vi "Parse DBL Array.vi"(6 "Seperator":string=",", 8 "error in":errorcluster, 9 "Input <JSON>":string, 10 "csv string":string, 11 "IParse CSV in":refnum<class "IParse CSV.lvclass">) -> (0 "error out":errorcluster, 2 "DBL Array":dbl[](array[numeric]), 3 "IParse CSV out":refnum<class "IParse CSV.lvclass">)   [LabVIEW 2024, in "IParse CSV.lvclass"]
uses:
  IParse CSV.lvclass
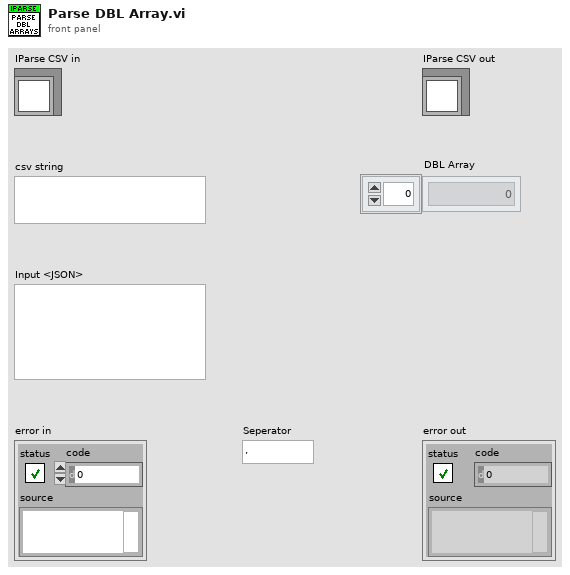
[diagram p1: front panel]
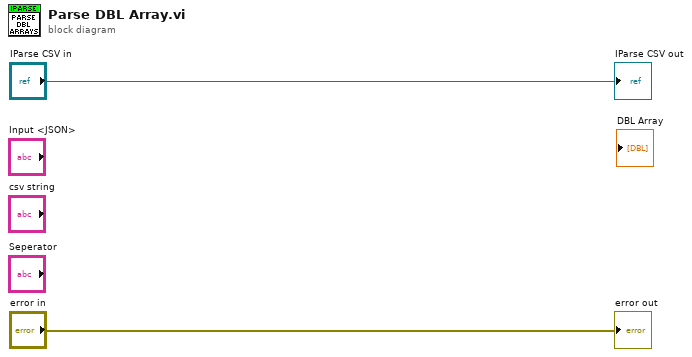
[diagram p0: block diagram]
diagram:
  "error out" <- "error in"
  "IParse CSV out" <- "IParse CSV in"
